vi "Handle setConfiguration.vi"(8 "error in (no error)":errorcluster, 10 "setConfiguration":variant, 11 "Instrument.Transport in":refnum<class "Inst.Transport.lvclass">) -> (0 "error out":errorcluster, 3 "Instrument.Transport out":refnum<class "Inst.Transport.lvclass">)   [LabVIEW 2019, in "Inst.Transport.lvclass"]
uses:
  Inst.Transport.lvclass
  3f43cf47-96c4-42eb-930c-20be6e2d6ff8.vi
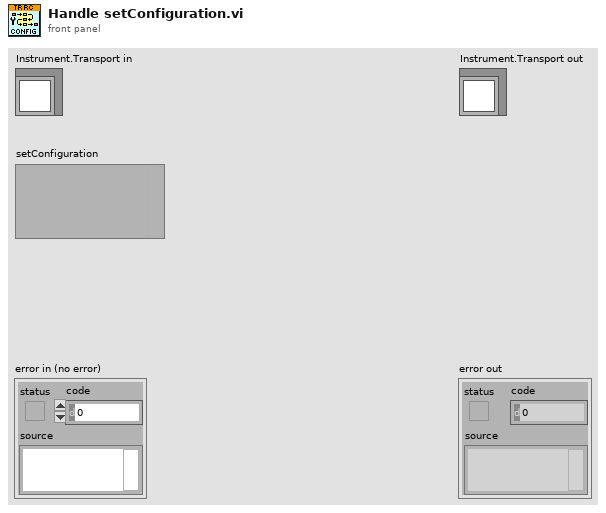
[diagram p1: front panel]
types:
  T1 = typedef "Inst.Transport.lvclass/Inst.Transport.Configuration--Cluster.ctl" = cluster{"Example Setting 1":dbl, "Example Setting 2":dbl, "Example Setting 3":string}
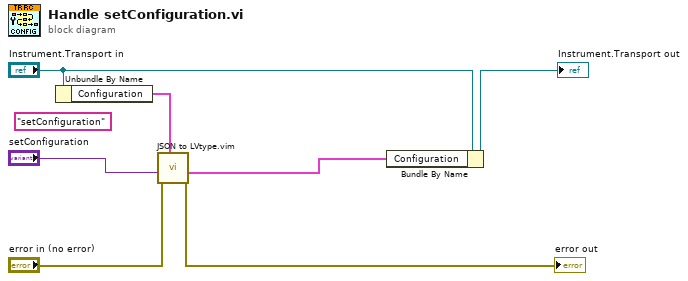
[diagram p0: block diagram]
diagram:
  (unwired) "setConfiguration" ("Command")
  n1 = Unbundle By Name("Instrument.Transport in") -> ("Configuration"=w1:T1)
  n2 = call "JSON to LVtype.vim"("type"=w1, "error in (no error)"="error in (no error)", "JSON Data in"="setConfiguration") -> ("error out"=→"error out":errorcluster, "Data out"=w5:T1)  [unwired: 7 in]
  n3 = Bundle By Name(cluster="Instrument.Transport in", "Configuration"=w5) -> (→"Instrument.Transport out":refnum<class "Inst.Transport.lvclass">)
